vi "pcfs_write_control_references.vi"(8 "error in (no error)":errorcluster, 10 "scan":refnum<vi>, 11 "scan_panel in":refnum<class "pcfs.lvclass">) -> (0 "error out":errorcluster, 3 "scan_panel out":refnum<class "pcfs.lvclass">)   [LabVIEW 2015, in "pcfs.lvclass"]
uses:
  pcfs.lvclass
  pcfs.lvclass/pcfs.ctl
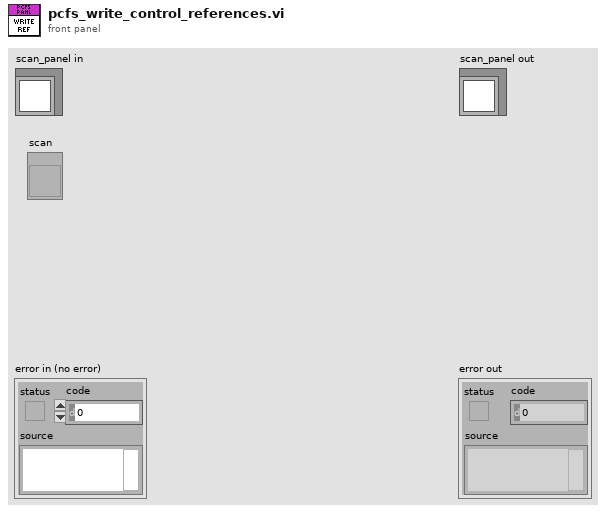
[diagram p1: front panel]
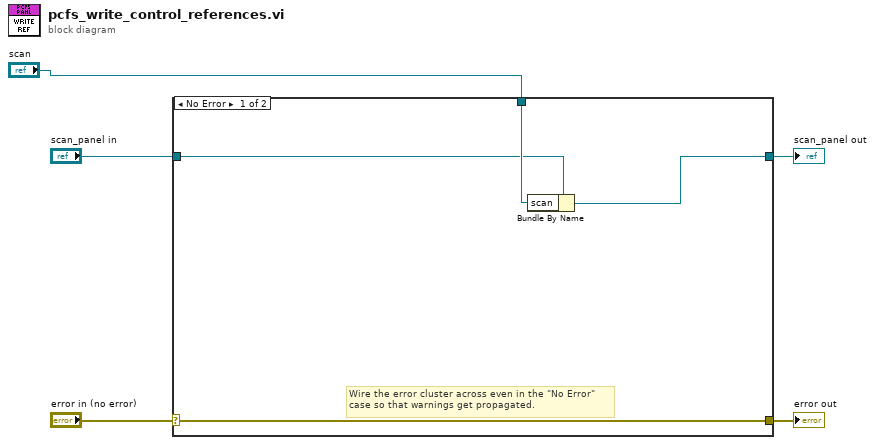
[diagram p0: block diagram]
diagram:
  n1 = case shown="No Error" "error in (no error)" {
    selector: "error in (no error)" -> [w9 w11]
    tunnel: [w9 w11] -> w4
    tunnel: [w6 w10] -> w2
    tunnel: "scan_panel in" -> [w7 w10]
    tunnel: "scan" -> [w8 _]
    frame No Error {
      # "Wire the error cluster across even in the \"No Error\"\ncase so that warnings get propagated."
      n2 = Bundle By Name(cluster=w7, "scan"=w8) -> (w6:refnum<class "pcfs.lvclass">)
    }
    frame Error {
    }
  }
  "error out" <- w4
  "scan_panel out" <- w2
